vi "TCP Check Connection.vi"(8 "error in (no error)":errorcluster, 11 "Connection In":T1) -> (0 "error out":errorcluster, 2 "Disconnected":bool, 3 "Connection out":T1)   [LabVIEW 2014, in "QwaveSys Raspberry Pi Library.lvlib"]
doc: "This VI removes the host connection from the connection manager list if it becomes disconnected for any reason."
uses:
  QwaveSys Raspberry Pi Library.lvlib
  TCP/stm_TCP Connection Info.ctl
  _SubVIs/stm_MetaDataElement.ctl
  stm_TCPConnectionMethod.ctl
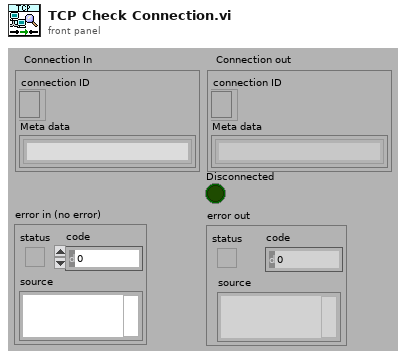
[diagram p1: front panel]
types:
  T1 = typedef "QwaveSys Raspberry Pi Library.lvlib/stm_TCP Connection Info.ctl" = cluster{"connection ID":refnum<k5>, "Meta data":T2[]}
  T2 = typedef "QwaveSys Raspberry Pi Library.lvlib/stm_MetaDataElement.ctl" = string
  T3 = typedef "QwaveSys Raspberry Pi Library.lvlib/stm_TCPConnectionMethod.ctl" = enum16{"Initialize", "Add Connection", "Set Properties", "Get Connection(s)", "Remove Connection", "Remove All Connections", "Get Connection Count"}
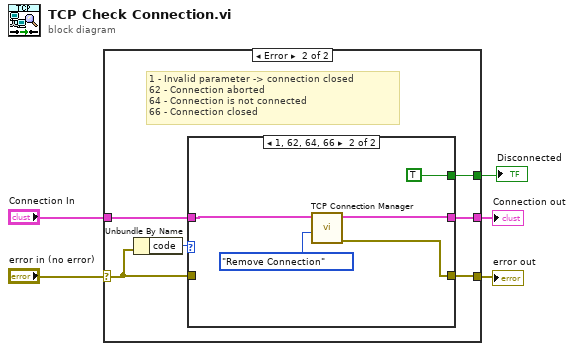
[diagram p0: block diagram]
diagram:
  n1 = case shown="Error" "error in (no error)" {
    selector: "error in (no error)" -> [w7 w12]
    tunnel: [w7 w11] -> w4
    tunnel: "Connection In" -> [w6 w10]
    tunnel: [w6 w9] -> w2
    tunnel: [_ w8] -> w1
    frame No Error {
    }
    frame Error {
      # "1 - Invalid parameter -> connection closed\n62 - Connection aborted\n64 - Connection is not connected\n66 - Connection closed"
      n2 = Unbundle By Name(w12) -> ("code"=w13:i32)
      n3 = case shown="1, 62, 64, 66" w13 {
        tunnel: w12 -> [w15 _]
        tunnel: [w15 w18] -> w11
        tunnel: w10 -> [w14 w17]
        tunnel: [w14 w16] -> w9
        tunnel: [_ TRUE] -> w8
        frame 0, Default {
        }
        frame 1, 62, 64, 66 {
          n4 = call "TCP Connection Manager.vi"("Method"=stm_TCPConnectionMethod."Remove Connection", "Connection In"=w17) -> ("error out"=w18:errorcluster, "Connection Out"=w16:T1)  [unwired: 3 in, 5 out]
        }
      }
    }
  }
  "error out" <- w4
  "Connection out" <- w2
  "Disconnected" <- w1
